vi "Calculate Receiver Sensitivity Threshold.vi"(11 "Packets to Generate":i32) -> (3 "Rx Sensitivity Threshold":i32)   [LabVIEW 2026, in "Nordic nRF52 DK DTM Test.lvlib"]
uses:
  Nordic nRF52 DK DTM Test.lvlib
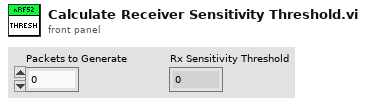
[diagram p1: front panel]
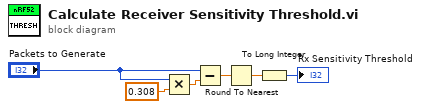
[diagram p0: block diagram]
diagram:
  n1 = Multiply(x="Packets to Generate", y=0.308) -> (x*y=w6:dbl)
  n2 = Subtract(x="Packets to Generate", y=w6) -> (x-y=w3:dbl)
  n3 = Round To Nearest(number=w3) -> (nearest integer value=w2:dbl)
  n4 = To Long Integer(number=w2) -> (32bit integer=→"Rx Sensitivity Threshold":i32)
